vi "Experimental.vi"   [LabVIEW 2018]
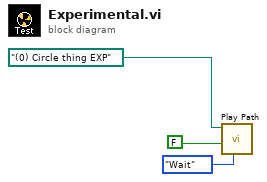
[diagram p0: block diagram]
diagram:
  n1 = call "Play Path.vi"("Synchronication"=enum16{"Start", "Wait"}."Wait", "Reverse (T) / Normal (F)"=FALSE ("Path Reversed"), "Path"=path "(0) Circle thing EXP") -> ()  [unwired: 8 in, 1 out]
